vi "Pre Launch Init.vi"(11 "CS++RTRootActor in":refnum<class "CS++RTRootActor.lvclass">) -> (0 "error out":errorcluster, 3 "CS++RTRootActor out":refnum<class "CS++RTRootActor.lvclass">)   [LabVIEW 2015, in "CS++RTRoot.lvlib" / "CS++RTRootActor.lvclass"]
doc: "(<B>Filename</B>: Actor Framework.lvlib:Actor.lvclass:Pre Launch Init.vi)\n\nDefines behavior that occurs after the Launch Nested Actor method is invoked but before the actor's Actor Core method begins running.\n\nBy default, this method does nothing. A descendant class may override it to define behavior."
uses:
  CS++RTRootActor.lvclass
  CSPP_Core/Classes/CS++BaseClasses/MessageLogger/CS++MessageLogger.lvclass
  CS++RTRootActor.lvclass/CS++RTRootActor.ctl
  CSPP_Core/Libraries/Base/Severity.ctl
  <vilib>/ActorFramework/Actor/Actor.lvclass
  CSPP_Core/Classes/CS++BaseClasses/Factory/CS++Factory.lvclass
  CSPP_Core/Libraries/Base/CS++Base.lvlib
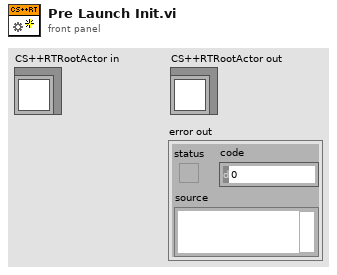
[diagram p1: front panel]
types:
  T1 = typedef "CS++Base.lvlib/Severity.ctl" = enum16{"emergency", "alert", "critical", "error", "warning", "notice", "info", "debug"}
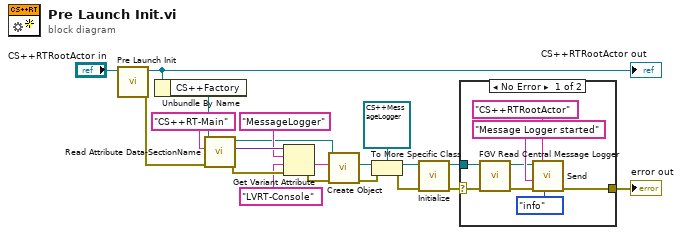
[diagram p0: block diagram]
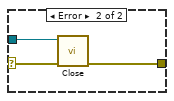
[diagram p2: hidden frame]
diagram:
  n1 = call-parent "Pre Launch Init.vi"("Actor in"="CS++RTRootActor in") -> ("error out"=w1:errorcluster, "Actor out"=w14:refnum<class "CS++RTRootActor.lvclass">)  [unwired: 9 in]
  "CS++RTRootActor out" <- w14
  n2 = Unbundle By Name(w14) -> ("CS++Factory"=w2:refnum<class "CS++Factory.lvclass">)
  n3 = call-dynamic "Read Attribute Data-SectionName.vi"("error in (no error)"=w1, "Object Name"="CS++RT-Main", "CS++Factory in"=w2) -> ("error out"=w11:errorcluster, "Attribute Data"=w12:variant, "CS++Factory out"=w6:refnum<class "CS++Factory.lvclass">)  [unwired: 6 in]
  n4 = Get Variant Attribute(Variant=w12, name="MessageLogger", default value (empty Variant)="LVRT-Console", error in=w11) -> (value=w7:string, error out=w8:errorcluster)  [unwired: 2 out]
  n5 = call "Create Object.vi"("error in (no error)"=w8, "Object Name"=w7, "CS++Factory in"=w6) -> ("error out"=w17:errorcluster, "LabVIEW Object"=w15:refnum<class>)  [unwired: 5 in, 2 out]
  n6 = To More Specific Class(target class=refnum<class "CS++MessageLogger.lvclass"> refnum ("CS++MessageLogger.lvlib:CS++MessageLogger.lvclass"), reference=w15, error in=w17) -> (specific class reference=w18:refnum<class "CS++MessageLogger.lvclass">, error out=w5:errorcluster)
  n7 = call "Initialize.vi"("Error In"=w5, "CS++MessageLogger in"=w18) -> ("Error Out"=w4:errorcluster, "CS++MessageLogger out"=w19:refnum<class "CS++MessageLogger.lvclass">)  [unwired: 8 in]
  n8 = case shown="No Error" w4 {
    selector: w4 -> [w23 w30]
    tunnel: w19 -> [w24 w31]
    tunnel: [w28 w29] -> w3
    frame No Error {
      n9 = call "FGV Read Central Message Logger.vi"("Error In"=w23, "CS++MessageLogger in"=w24) -> ("Error Out"=w21:errorcluster, "CS++MessageLogger out"=w22:refnum<class "CS++MessageLogger.lvclass">)  [unwired: 8 in]
      n10 = call "Send.vi"("Severity Code (info)"=Severity."info", "Error In"=w21, "Message Content"="Message Logger started", "Message Tag"="CS++RTRootActor", "CS++MessageLogger in"=w22) -> ("Error Out"=w28:errorcluster)  [unwired: 5 in, 1 out]
    }
    frame Error {
      n11 = call "Close.vi"("Error In"=w30, "CS++MessageLogger in"=w31) -> ("Error Out"=w29:errorcluster)  [unwired: 8 in, 1 out]
    }
  }
  "error out" <- w3
